vi "WPI_Get Camera Dev Ref Notifier.vi"(8 "error in (no error)":errorcluster, 11 "Camera Address":string) -> (0 "error out":errorcluster, 3 "notifier out":refnum<notifier>)   [LabVIEW 2017]
doc: "This software is licensed. Open the labview\\readme\\WPI Robotics Library Open Source License.txt file for more information."
uses:
  <vilib>/Rock Robotics/WPI/Camera/WPI_CameraDevRef.ctl
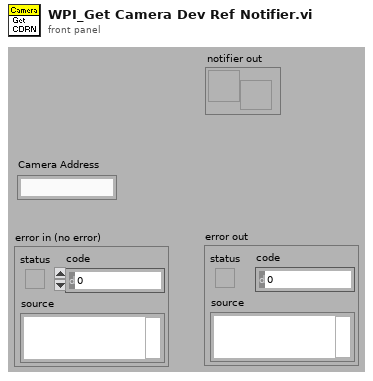
[diagram p1: front panel]
types:
  T1 = typedef "WPI_CameraDevRef.ctl" = cluster{"Camera Address":string, "CameraStatus":errorcluster}
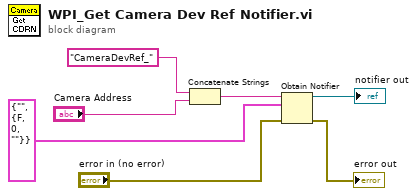
[diagram p0: block diagram]
diagram:
  n1 = Concatenate Strings("CameraDevRef_" ("format string"), "Camera Address") -> (w7:string)
  n2 = Obtain Notifier(name (unnamed)=w7, notification data type=T1 {"Camera Address"="", "CameraStatus"={"status"=FALSE, "code"=0, "source"=""}} ("CameraDevRef"), error in (no error)="error in (no error)") -> (notifier out=→"notifier out":refnum<notifier>, error out=→"error out":errorcluster)  [unwired: 1 in, 1 out]
